vi "GSP_Logger.vi"() -> ()   [LabVIEW 2015]
uses:
  LoggerParameters.ctl
  <vilib>/Utility/error.llb/DialogType.ctl
  LogItem.ctl
  GSP_Logger_Global.vi
  GUI/GSP_GUI_global.vi
panel:
  out "Error Message":string
  in  "Logger Parameters":T1
  in  "Past Events":i32(listbox)
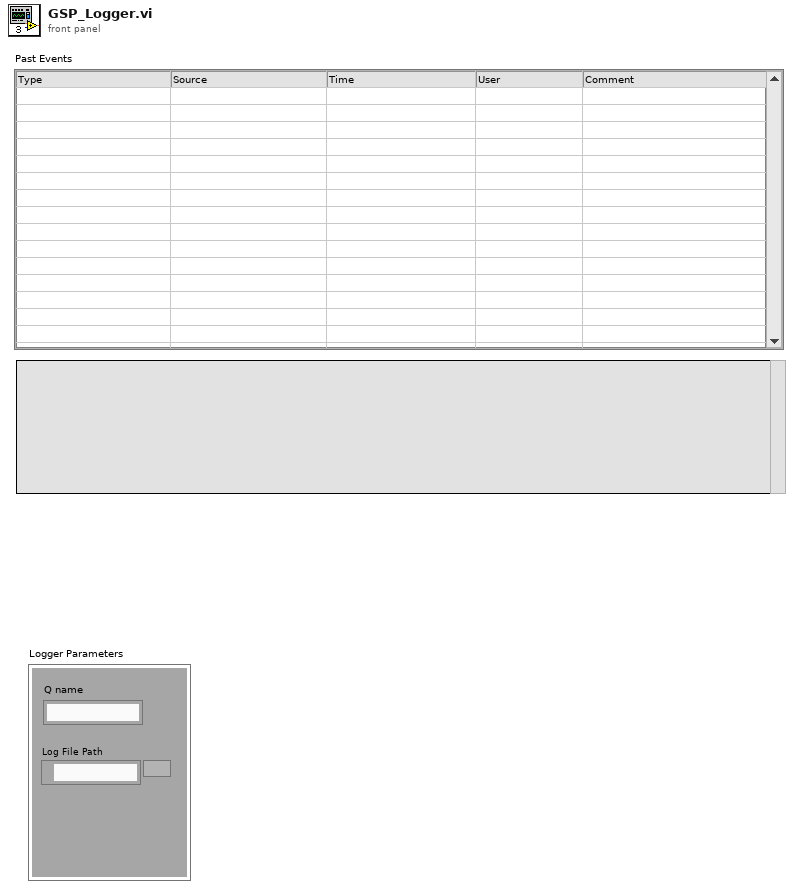
[diagram p1: front panel]
types:
  T1 = typedef "LoggerParameters.ctl" = cluster{"Q name":string, "Log File Path":path}
  T2 = cluster{"error in (no error)":errorcluster, "Source":string, "Comment":string, "current time":timestamp, "user":string}[]
  T3 = enum16{"Launch", "Log", "Open", "Close", "Shutdown"}
  T4 = cluster{"error in (no error)":errorcluster, "Source":string, "Comment":string, "current time":timestamp, "user":string}
  T5 = typedef "LogItem.ctl" = cluster{"error in (no error)":errorcluster, "Source":string, "Comment ":string}
  T6 = typedef "DialogType.ctl" = u16
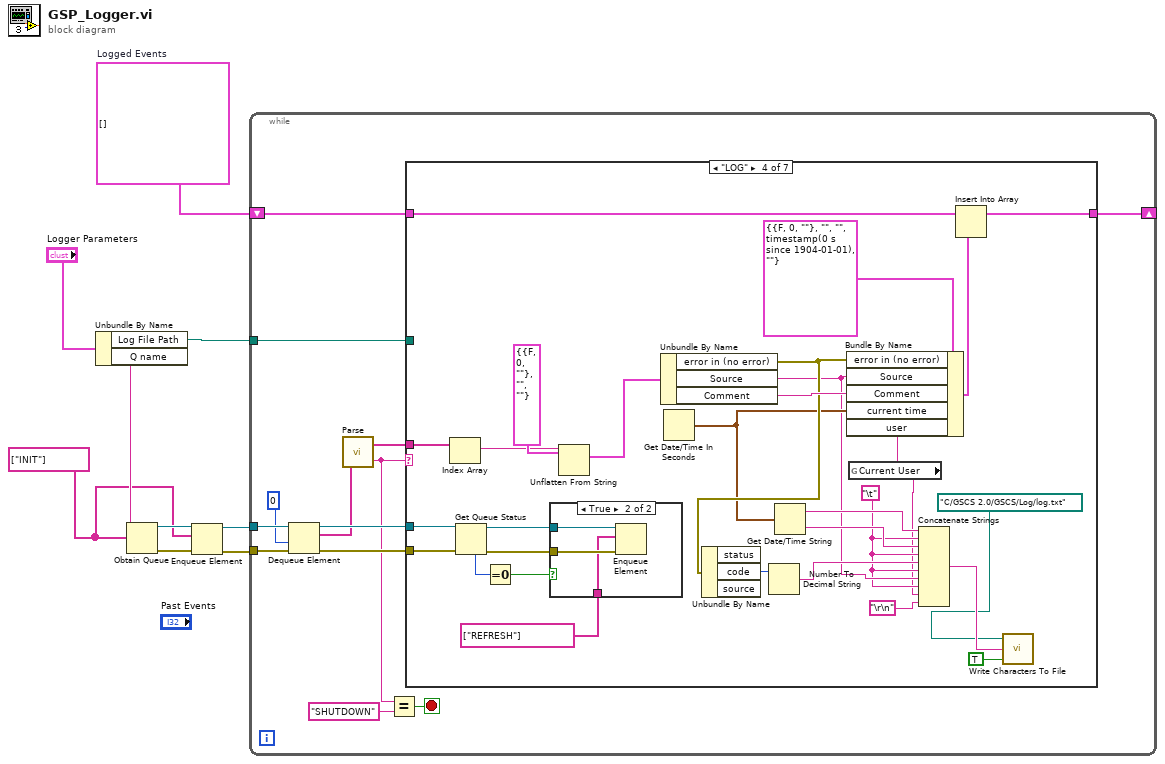
[diagram p0: block diagram]
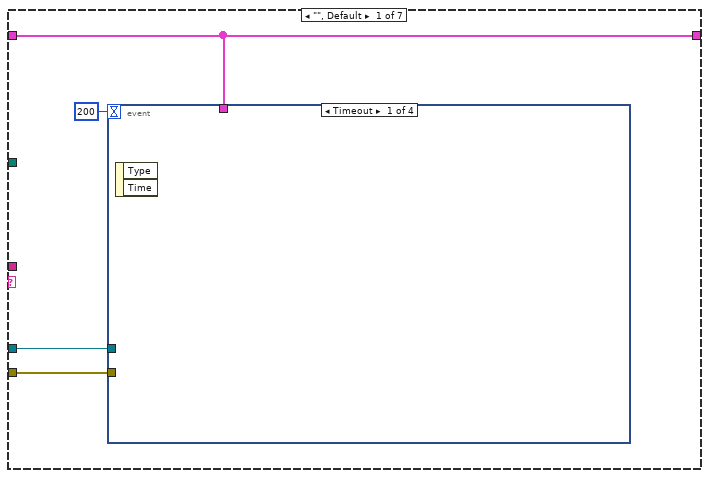
[diagram p2: hidden frame]
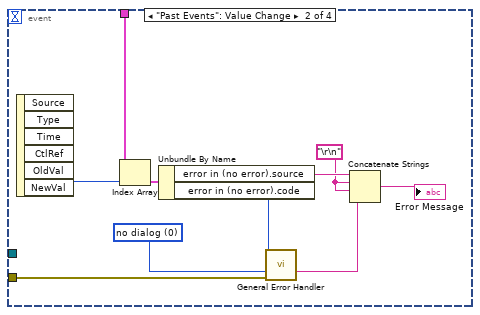
[diagram p3: hidden frame]
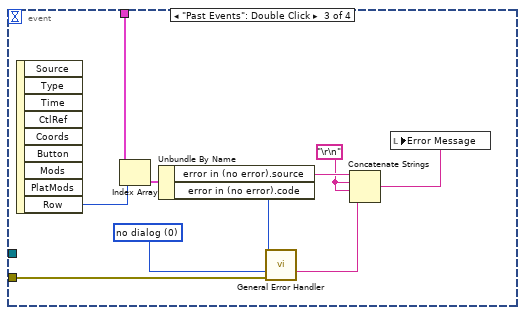
[diagram p4: hidden frame]
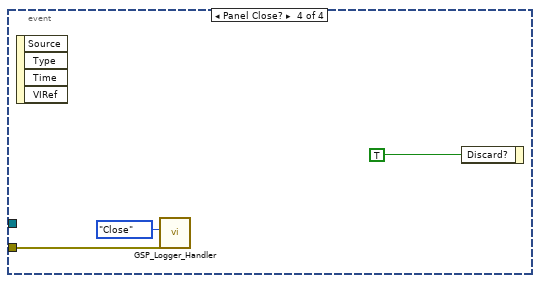
[diagram p5: hidden frame]
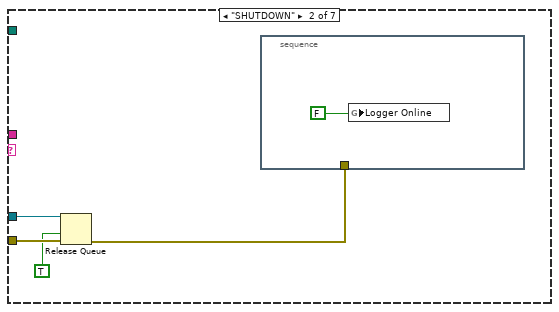
[diagram p6: hidden frame]
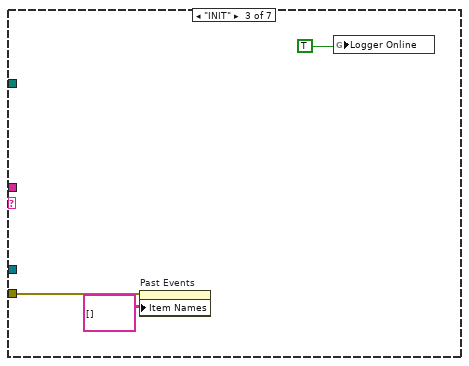
[diagram p7: hidden frame]
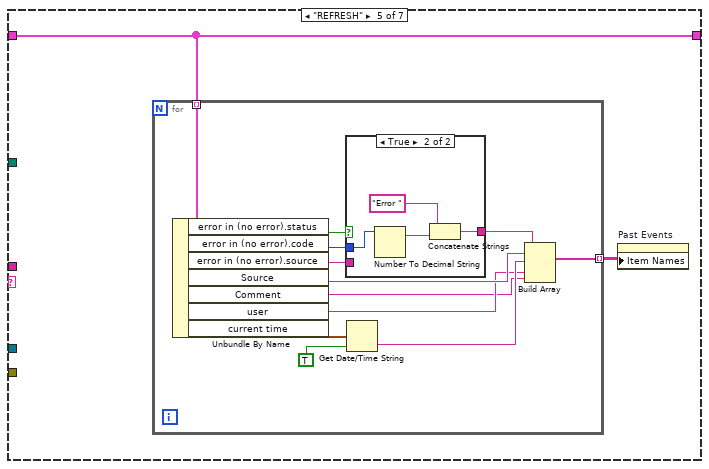
[diagram p9: hidden frame]
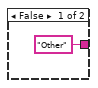
[diagram p10: hidden frame]
diagram:
  w1 = T2 []  # Logged Events
  w2 = string[] ["INIT"] ("element")
  n1 = Unbundle By Name("Logger Parameters") -> ("Log File Path"=w6:path, "Q name"=w3:string)
  n2 = Obtain Queue(name (unnamed)=w3, element data type=w2) -> (queue out=w5:refnum<queue>, error out=w4:errorcluster)  [unwired: 3 in, 1 out]
  n3 = Enqueue Element(queue=w5, element=w2, error in (no error)=w4) -> (queue out=w8:refnum<queue>, error out=w9:errorcluster)  [unwired: 1 in, 1 out]
  n4 = while {
    tunnel: w9 -> [w20]
    tunnel: w8 -> [w21]
    tunnel: w6 -> [w22]
    shift-right: [w11] -> _
    shift-left: w1 -> [w12]
    stop <- w16 stop-if-true
    n5 = Dequeue Element(queue=w21, timeout in ms (-1)=0, error in (no error)=w20) -> (queue out=w18:refnum<queue>, element=w13:string[], error out=w17:errorcluster)  [unwired: 1 out]
    n6 = call "Parse.vi"("Command Array"=w13) -> ("Parameters"=w19:string[], "Command"=w15:string)
    n7 = Equal?(x=w15, y="SHUTDOWN") -> (x = y?=w16:bool)
    n8 = case shown="\"LOG\"" w15 {
      tunnel: w22 -> [_ _ _ _ _ _ _]
      tunnel: w19 -> [_ _ _ w86 _ _ _]
      tunnel: w18 -> [w25 w53 _ w78 _ _ _]
      tunnel: w17 -> [w26 w52 w56 w77 _ _ _]
      tunnel: w12 -> [w24 _ _ w83 w91 w109 w110]
      tunnel: [w24 _ _ w79 w91 w109 w110] -> w11
      frame "", Default {
        n9 = event shown="[0] Timeout" {
          selector: _ -> [_ _ _ _]
          dyn-events: _ -> [_ _ _ _]
          timeout: 200 -> [_ _ _ _]
          tunnel: w26 -> [_ w32 w43 w48]
          tunnel: w25 -> [_ _ _ _]
          tunnel: w24 -> [_ w36 w46 _]
          event Timeout {
            n10 = event-data() -> ()  [unwired: 1 in, 2 out]
          }
          event "Past Events": Value Change {
            w33 = T6 0 items=["no dialog", "OK message", "continue or stop message", "OK message + warnings", "continue/stop + warnings"] ("type of dialog (OK msg:1)")
            w27 = "\r\n"
            n11 = event-data() -> ("NewVal"=w35:i32)  [unwired: 1 in, 5 out]
            n12 = Index Array(array=w36, index=w35) -> (element=w34:T4)
            n13 = Unbundle By Name(w34) -> ("error in (no error).source"=w30:string, "error in (no error).code"=w31:i32)
            n14 = call <vilib>:"General Error Handler.vi"("[error code] (0)"=w31, "type of dialog (OK msg:1)"=w33, "error in (no error)"=w32) -> ("message"=w29:string)  [unwired: 8 in, 4 out]
            n15 = Concatenate Strings(w30, w27, w27, w29) -> (→"Error Message":string)
          }
          event "Past Events": Double Click {
            w44 = T6 0 items=["no dialog", "OK message", "continue or stop message", "OK message + warnings", "continue/stop + warnings"] ("type of dialog (OK msg:1)")
            w39 = "\r\n"
            n16 = event-data() -> ("Row"=w37:i32)  [unwired: 1 in, 8 out]
            n17 = Index Array(array=w46, index=w37) -> (element=w45:T4)
            n18 = Unbundle By Name(w45) -> ("error in (no error).source"=w41:string, "error in (no error).code"=w42:i32)
            n19 = call <vilib>:"General Error Handler.vi"("[error code] (0)"=w42, "type of dialog (OK msg:1)"=w44, "error in (no error)"=w43) -> ("message"=w40:string)  [unwired: 8 in, 4 out]
            n20 = Concatenate Strings(w41, w39, w39, w40) -> (w38:string)
            n21 = local write "Error Message"(w38) -> ()
          }
          event Panel Close? {
            n22 = event-data() -> ()  [unwired: 1 in, 4 out]
            n23 = call "GSP_Logger_Handler.vi"("error in (no error)"=w48, "Actions"=T3."Close") -> ()  [unwired: 5 in, 1 out]
            n24 = event-data("Discard?"=TRUE) -> ()  [unwired: 1 in, 1 out]
          }
        }
      }
      frame "SHUTDOWN" {
        n25 = Release Queue(queue=w53, force destroy? (F)=TRUE, error in (no error)=w52) -> (error out=w51:errorcluster)  [unwired: 2 out]
        n26 = stacked-sequence {
          tunnel: w51 -> [_]
          frame #0 {
            n27 = global write "GSP_Logger_Global.vi" "Logger Online"(FALSE) -> ()
          }
        }
      }
      frame "INIT" {
        n28 = property on="Past Events" class="MCListbox (strict)"(error in=w56, "Item Names"=string[][] []) -> ()  [unwired: 1 in, 2 out]
        n29 = global write "GSP_Logger_Global.vi" "Logger Online"(TRUE) -> ()
      }
      frame "LOG" {
        w62 = "\t"
        n30 = Index Array(array=w86) -> (element=w84:string)  [unwired: 1 in]
        n31 = Get Queue Status(queue=w78, error in (no error)=w77) -> (queue out=w76:refnum<queue>, error out=w75:errorcluster, # elements in queue=w74:i32)  [unwired: 1 in, 5 out]
        n32 = Equal To 0?(x=w74) -> (x = 0?=w73:bool)
        n33 = case shown="True" w73 {
          tunnel: w76 -> [_ w89]
          tunnel: w75 -> [_ w88]
          tunnel: string[] ["REFRESH"] ("element") -> [_ w87]
          frame False {
          }
          frame True {
            n34 = Enqueue Element(queue=w89, element=w87, error in (no error)=w88) -> ()  [unwired: 1 in, 3 out]
          }
        }
        n35 = Unflatten From String(type=T5 {"error in (no error)"={"status"=FALSE, "code"=0, "source"=""}, "Source"="", "Comment "=""} ("Log"), binary string=w84) -> (value=w81:T5)  [unwired: 3 in, 2 out]
        n36 = Unbundle By Name(w81) -> ("error in (no error)"=w70:errorcluster, "Source"=w63:string, "Comment"=w80:string)
        n37 = Get Date/Time In Seconds() -> (seconds since 1Jan1904=w67:timestamp)
        n38 = Unbundle By Name(w70) -> ("code"=w68:i32)  [unwired: 2 out]
        n39 = Number To Decimal String(number=w68) -> (decimal integer string=w64:string)  [unwired: 1 in]
        n40 = Get Date/Time String(seconds (now)=w67) -> (date string=w66:string, time string=w65:string)  [unwired: 2 in]
        n41 = global read "GSP_GUI_global.vi" "Current User"() -> (w61:string)
        n42 = Bundle By Name(cluster=T4 {"error in (no error)"={"status"=FALSE, "code"=0, "source"=""}, "Source"="", "Comment"="", "current time"=timestamp(0 s since 1904-01-01), "user"=""} ("Logged Events"), "error in (no error)"=w70, "Source"=w63, "Comment"=w80, "current time"=w67, "user"=w61) -> (w71:T4)
        n43 = Concatenate Strings(w66, w62, w65, w62, w64, w62, w63, w62, w61, "\r\n") -> (w60:string)
        n44 = Insert Into Array(array=w83, new element=w71) -> (w79:T2)  [unwired: 1 in]
        n45 = call <vilib>:"Write Characters To File.vi"("append to file? (new file:F)"=TRUE, "character string"=w60, "file path (dialog if empty)"=path "C:/GSCS 2.0/GSCS/Log/log.txt") -> ()  [unwired: 2 in, 1 out]
      }
      frame "REFRESH" {
        n46 = for {
          tunnel: w91 -> [w103] mode=indexing
          tunnel: [w97] -> w90 mode=indexing
          n47 = Unbundle By Name(w103) -> ("error in (no error).status"=w102:bool, "error in (no error).code"=w93:i32, "error in (no error).source"=w92:string, "Source"=w99:string, "Comment"=w94:string, "user"=w95:string, "current time"=w96:timestamp)
          n48 = case shown="True" w102 {
            tunnel: w93 -> [_ w108]
            tunnel: ["Other" w105] -> w100
            tunnel: w92 -> [_ _]
            frame False {
            }
            frame True {
              n49 = Number To Decimal String(number=w108) -> (decimal integer string=w106:string)  [unwired: 1 in]
              n50 = Concatenate Strings("Error ", w106) -> (w105:string)
            }
          }
          n51 = Get Date/Time String(seconds (now)=w96, want seconds? (F)=TRUE) -> (time string=w98:string)  [unwired: 1 in, 1 out]
          n52 = Build Array(w100, w99, w98, w95, w94) -> (w97:string[])
        }
        n53 = property on="Past Events" class="MCListbox (strict)"("Item Names"=w90) -> ()  [unwired: 2 in, 2 out]
      }
      frame "OPEN" {
      }
      frame "CLOSE" {
      }
    }
  }
